vi "Slider Set Limit.vi"(6 "Lower/Upper":T1, 8 "Value":dbl, 9 "Index":i32, 10 "LBCB Number":T2, 11 "DofType":T3) -> ()   [LabVIEW 2009]
uses:
  Data Access Objects/Limits/DofTypes.ctl
  Data Access Objects/Metadata/LBCB Number.ctl
  Lower Upper Select.ctl
  Data Access Objects/Metadata/Persistant DAO Actions.ctl
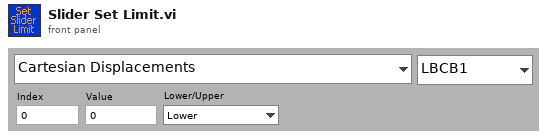
[diagram p1: front panel]
types:
  T1 = typedef "Lower Upper Select.ctl" = enum16{"Lower", "Upper"}
  T2 = typedef "LBCB Number.ctl" = enum16{"LBCB1", "LBCB2"}
  T3 = typedef "DofTypes.ctl" = enum16{"Cartesian Displacements", "Cartesian Forces & Moments", "Actuator Displacements", "Actuator Forces"}
  T4 = typedef "Persistant DAO Actions.ctl" = enum16{"Init", "Get", "Set", "Load", "Save"}
  T5 = typedef "Cartesian Matrix.ctl" = cluster{"Lower":T6, "Upper":T6}
  T6 = typedef "Cartesian Point.ctl" = cluster{"Dx":dbl, "Dy":dbl, "Dz":dbl, "Rx":dbl, "Ry":dbl, "Rz":dbl}
  T7 = typedef "Limit Matrix.ctl" = dbl[][]
  T8 = typedef "Actuator Matrix.ctl" = cluster{"Lower":T9, "Upper":T9}
  T9 = typedef "Actuator Point.ctl" = cluster{"X1":dbl, "X2":dbl, "Y1":dbl, "Z1":dbl, "Z2":dbl, "Z3":dbl}
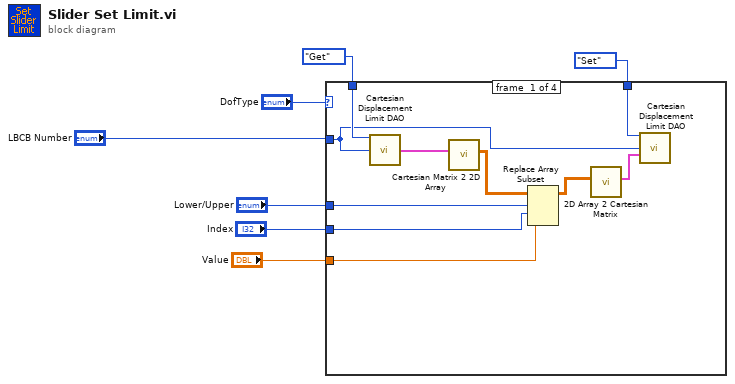
[diagram p0: block diagram]
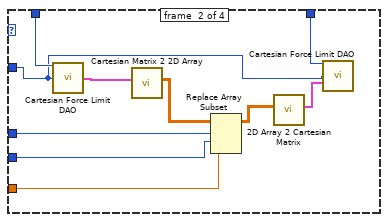
[diagram p2: hidden frame]
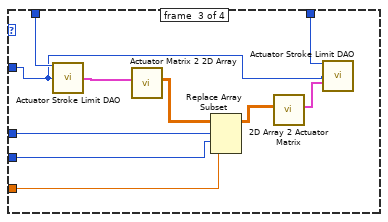
[diagram p3: hidden frame]
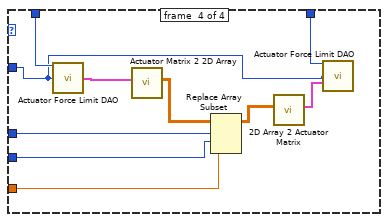
[diagram p4: hidden frame]
diagram:
  n1 = case shown="\"Cartesian Displacements\"" "DofType" {
    tunnel: Persistant_DAO_Actions."Get" ("Cartesian Displacement Limit Actions") -> [w17 w27 w37 w47]
    tunnel: "LBCB Number" -> [w14 w24 w34 w44]
    tunnel: Persistant_DAO_Actions."Set" ("Cartesian Displacement Limit Actions") -> [w15 w25 w35 w45]
    tunnel: "Lower/Upper" -> [w12 w22 w32 w42]
    tunnel: "Index" -> [w11 w21 w31 w41]
    tunnel: "Value" -> [w10 w20 w30 w40]
    frame #0 {
      n2 = call "Cartesian Displacement Limit DAO.vi"("Cartesian Displacement Limit Actions"=w17, "ID"=w14) -> ("Cartesian Displacement Out"=w16:T5)  [unwired: 11 in, 2 out]
      n3 = call "Cartesian Matrix 2 2D Array.vi"("Matrix In"=w16) -> ("Matrix Out"=w13:T7)  [unwired: 10 in]
      n4 = Replace Array Subset(array=w13, new element=w10, index (row)=w12, index (col)=w11) -> (w9:T7)
      n5 = call "2D Array 2 Cartesian Matrix.vi"("Matrix In"=w9) -> ("Matrix Out"=w8:T5)  [unwired: 10 in]
      n6 = call "Cartesian Displacement Limit DAO.vi"("Cartesian Displacement Limit Actions"=w15, "ID"=w14, "Cartesian Displacement In"=w8) -> ()  [unwired: 10 in, 3 out]
    }
    frame #1 {
      n7 = call "Cartesian Force Limit DAO.vi"("Cartesian Force Limit Actions"=w27, "ID"=w24) -> ("Cartesian Force Limit Out"=w26:T5)  [unwired: 11 in, 2 out]
      n8 = call "Cartesian Matrix 2 2D Array.vi"("Matrix In"=w26) -> ("Matrix Out"=w23:T7)  [unwired: 10 in]
      n9 = Replace Array Subset(array=w23, new element=w20, index (row)=w22, index (col)=w21) -> (w19:T7)
      n10 = call "2D Array 2 Cartesian Matrix.vi"("Matrix In"=w19) -> ("Matrix Out"=w18:T5)  [unwired: 10 in]
      n11 = call "Cartesian Force Limit DAO.vi"("Cartesian Force Limit Actions"=w25, "ID"=w24, "Cartesian Force Limit In"=w18) -> ()  [unwired: 10 in, 3 out]
    }
    frame #2 {
      n12 = call "Actuator Stroke Limit DAO.vi"("Actuator Stroke Limit Actions"=w37, "ID"=w34) -> ("Actuator Stroke Limits Out"=w36:T8)  [unwired: 11 in, 2 out]
      n13 = call "Actuator Matrix 2 2D Array.vi"("Matrix In"=w36) -> ("Matrix Out"=w33:T7)  [unwired: 10 in]
      n14 = Replace Array Subset(array=w33, new element=w30, index (row)=w32, index (col)=w31) -> (w29:T7)
      n15 = call "2D Array 2 Actuator Matrix.vi"("Matrix In"=w29) -> ("Matrix Out"=w28:T8)  [unwired: 10 in]
      n16 = call "Actuator Stroke Limit DAO.vi"("Actuator Stroke Limit Actions"=w35, "ID"=w34, "Actuator Stroke Limits In"=w28) -> ()  [unwired: 10 in, 3 out]
    }
    frame #3 {
      n17 = call "Actuator Force Limit DAO.vi"("Actuator Force Limit Actions"=w47, "ID"=w44) -> ("Actuator Force Limits Out"=w46:T8)  [unwired: 11 in, 2 out]
      n18 = call "Actuator Matrix 2 2D Array.vi"("Matrix In"=w46) -> ("Matrix Out"=w43:T7)  [unwired: 10 in]
      n19 = Replace Array Subset(array=w43, new element=w40, index (row)=w42, index (col)=w41) -> (w39:T7)
      n20 = call "2D Array 2 Actuator Matrix.vi"("Matrix In"=w39) -> ("Matrix Out"=w38:T8)  [unwired: 10 in]
      n21 = call "Actuator Force Limit DAO.vi"("Actuator Force Limit Actions"=w45, "ID"=w44, "Actuator Force Limits  Input"=w38) -> ()  [unwired: 10 in, 3 out]
    }
  }
